vi "Register Dynamic Events.vi"(8 "error in (no error)":errorcluster, 11 "ApplicationEventHandler In":refnum<class "ApplicationEventHandler.lvclass">) -> (0 "error out":errorcluster, 3 "ApplicationEventHandler Out":refnum<class "ApplicationEventHandler.lvclass">)   [LabVIEW 2015, in "ActorEvents.lvlib" / "ApplicationEventHandler.lvclass"]
uses:
  ApplicationEventHandler.lvclass
  IEventHandler/IEventHandler.lvclass/IEventHandler.ctl
  ApplicationEventHandler.lvclass/ApplicationEventHandler.ctl
  IEventHandler/IEventHandler.lvclass
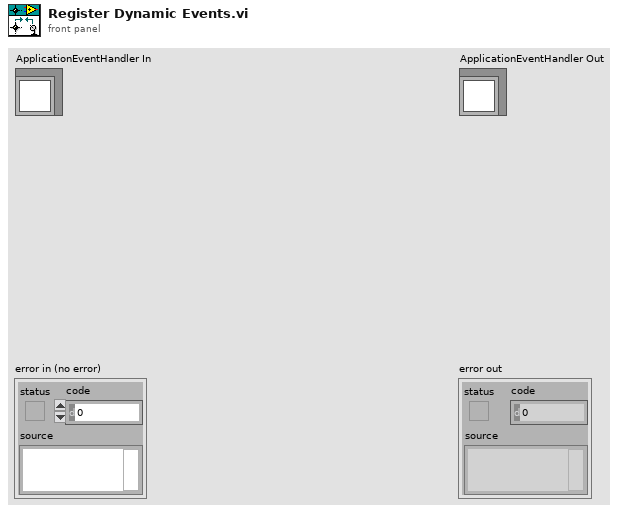
[diagram p1: front panel]
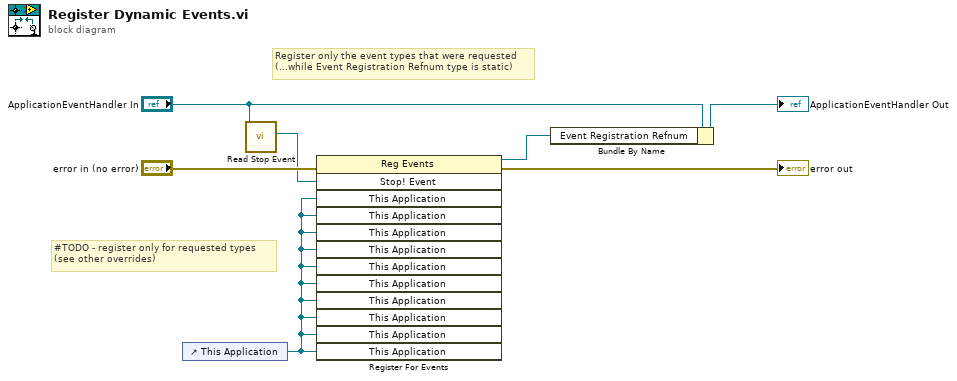
[diagram p0: block diagram]
diagram:
  # "#TODO - register only for requested types\n(see other overrides)"
  # "Register only the event types that were requested\n(...while Event Registration Refnum type is static)"
  n1 = control-ref of="This Application"() -> (w7:refnum<vi>)
  n2 = call "Read Stop Event.vi"("IEventHandler in"="ApplicationEventHandler In") -> ("Stop! Event"=w2:refnum<user-event>)  [unwired: 10 in]
  n3 = register-events(error in="error in (no error)", w2, w7, w7, w7, w7, w7, w7, w7, w7, w7, w7) -> (reference out=w1:refnum<event-registration>, error out=→"error out":errorcluster)  [unwired: 1 in]
  n4 = Bundle By Name(cluster="ApplicationEventHandler In", "Event Registration Refnum"=w1) -> (→"ApplicationEventHandler Out":refnum<class "ApplicationEventHandler.lvclass">)
